vi "Step x0.5.vi"(8 "error in (no error)":errorcluster, 11 "Measurement2D in":refnum<class "Measurement2D.lvclass">) -> (0 "error out":errorcluster, 3 "Measurement2D out":refnum<class "Measurement2D.lvclass">)   [LabVIEW 2018, in "Measurement2D.lvclass"]
uses:
  Measurement2D.lvclass
  Measurement2D.lvclass/Measurement2D.ctl
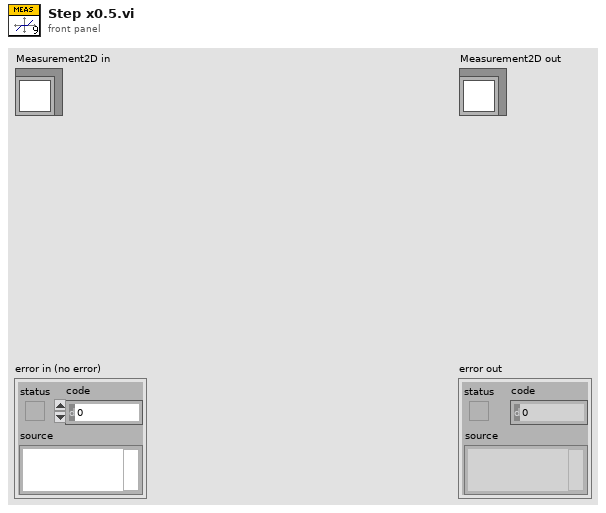
[diagram p1: front panel]
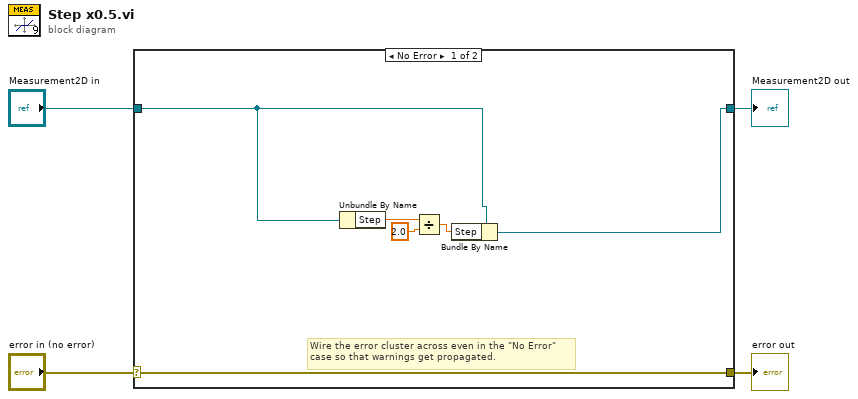
[diagram p0: block diagram]
diagram:
  n1 = case shown="No Error" "error in (no error)" {
    selector: "error in (no error)" -> [w10 w12]
    tunnel: [w10 w12] -> w3
    tunnel: [w5 w11] -> w1
    tunnel: "Measurement2D in" -> [w6 w11]
    frame No Error {
      # "Wire the error cluster across even in the \"No Error\"\ncase so that warnings get propagated."
      n2 = Unbundle By Name(w6) -> ("Step"=w8:dbl)
      n3 = Divide(x=w8, y=2.0 ("x")) -> (x/y=w9:dbl)
      n4 = Bundle By Name(cluster=w6, "Step"=w9) -> (w5:refnum<class "Measurement2D.lvclass">)
    }
    frame Error {
    }
  }
  "error out" <- w3
  "Measurement2D out" <- w1
